vi "test for loop com.vi"() -> ()   [LabVIEW 2010]
panel:
  out "com transpose":dbl
  out "com":dbl
  in  "2d array":u16[][](array[numeric])
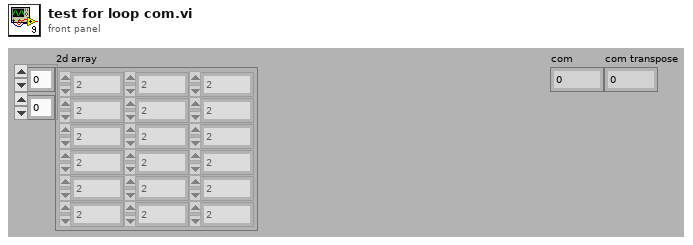
[diagram p1: front panel]
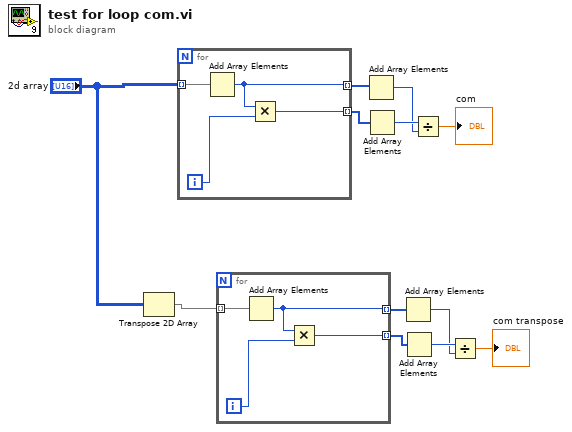
[diagram p0: block diagram]
diagram:
  n1 = Transpose 2D Array(2D array="2d array") -> (transposed array=w6:u16[][])
  n2 = for {
    tunnel: "2d array" -> [w16] mode=indexing
    tunnel: [w15] -> w12 mode=indexing
    tunnel: [w13] -> w11 mode=indexing
    i -> [w14]
    n3 = Add Array Elements(numeric array=w16) -> (sum=w15:u16)
    n4 = Multiply(x=w15, y=w14) -> (x*y=w13:i32)
  }
  n5 = for {
    tunnel: w6 -> [w20] mode=indexing
    tunnel: [w19] -> w3 mode=indexing
    tunnel: [w17] -> w2 mode=indexing
    i -> [w18]
    n6 = Add Array Elements(numeric array=w20) -> (sum=w19:u16)
    n7 = Multiply(x=w19, y=w18) -> (x*y=w17:i32)
  }
  n8 = Add Array Elements(numeric array=w12) -> (sum=w9:u16)
  n9 = Add Array Elements(numeric array=w11) -> (sum=w10:i32)
  n10 = Add Array Elements(numeric array=w3) -> (sum=w4:u16)
  n11 = Add Array Elements(numeric array=w2) -> (sum=w5:i32)
  n12 = Divide(x=w10, y=w9) -> (x/y=→"com":dbl)
  n13 = Divide(x=w5, y=w4) -> (x/y=→"com transpose":dbl)
